vi "DPO_7K_Default Settings.vi"(8 "Error In":errorcluster, 11 "VISA resource name in":refnum<visa-resource-name>) -> (0 "error out":errorcluster, 3 "VISA resource name out":refnum<visa-resource-name>)   [LabVIEW 2020]
doc: "Establishes communication with the instrument and optionally performs an instrument identification query or an instrument reset. This VI also places the instrument in a default state needed for other instrument driver operations.\nRun this VI before running other instrument driver VIs for the instrument. You generally need to run the Initialize VI only once, at the beginning of an application."
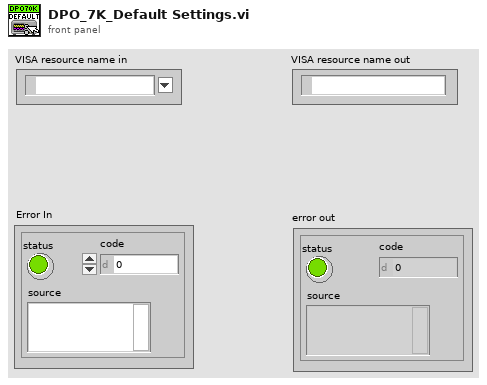
[diagram p1: front panel]
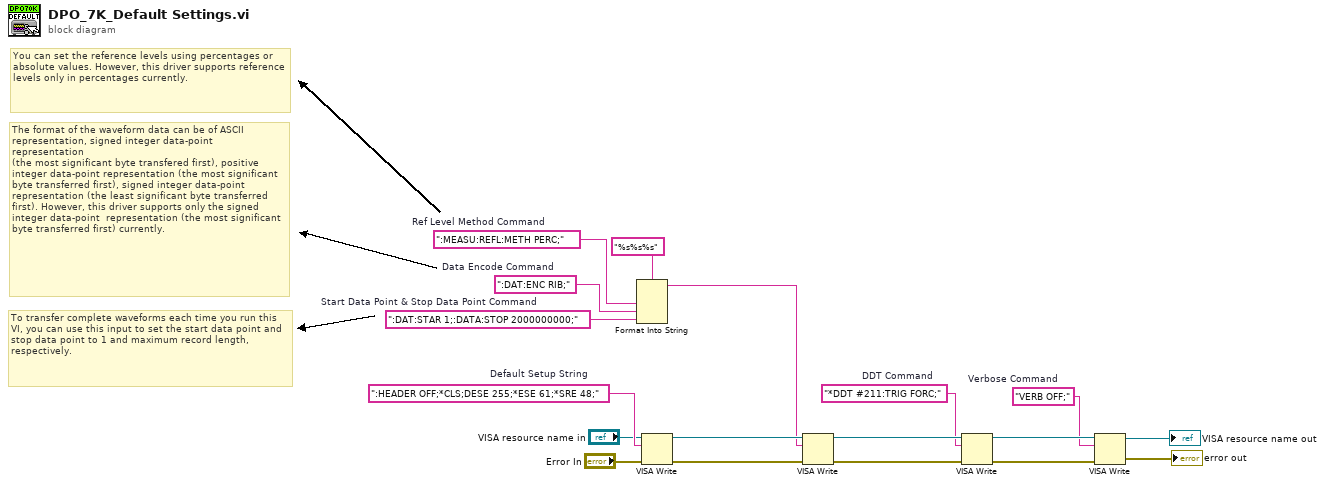
[diagram p0: block diagram]
diagram:
  w5 = ":DAT:STAR 1;:DATA:STOP 2000000000;"  # Start Data Point & Stop Data Point Command
  w6 = ":DAT:ENC RIB;"  # Data Encode Command
  w7 = ":HEADER OFF;*CLS;DESE 255;*ESE 61;*SRE 48;"  # Default Setup String
  w8 = "VERB OFF;"  # Verbose Command
  w11 = "*DDT #211:TRIG FORC;"  # DDT Command
  w18 = ":MEASU:REFL:METH PERC;"  # Ref Level Method Command
  # "To transfer complete waveforms each time you run this VI, you can use this input to set the start data point and stop data point to 1 and maximum record length, respectively."
  # "The format of the waveform data can be of ASCII\nrepresentation, signed integer data-point representation \n(the most significant byte transfered first), positive \ninteger data-point representation (the most significant \nbyte transferred first), signed integer data-point \nrepresentation (the least significant byte transferred first). However, this driver supports only the signed integer data-point  representation (the most significant byte transferred first) currently."
  # "You can set the reference levels using percentages or absolute values. However, this driver supports reference levels only in percentages currently."
  n1 = Format Into String(format string="%s%s%s", w18, w6, w5) -> (resulting string=w15:string)  [unwired: 2 in, 1 out]
  n2 = VISA Write(VISA resource name="VISA resource name in", write buffer=w7, error in (no error)="Error In") -> (VISA resource name out=w17:refnum<visa-resource-name>, error out=w16:errorcluster)  [unwired: 1 out]
  n3 = VISA Write(VISA resource name=w17, write buffer=w15, error in (no error)=w16) -> (VISA resource name out=w13:refnum<visa-resource-name>, error out=w12:errorcluster)  [unwired: 1 out]
  n4 = VISA Write(VISA resource name=w13, write buffer=w11, error in (no error)=w12) -> (VISA resource name out=w10:refnum<visa-resource-name>, error out=w9:errorcluster)  [unwired: 1 out]
  n5 = VISA Write(VISA resource name=w10, write buffer=w8, error in (no error)=w9) -> (VISA resource name out=→"VISA resource name out":refnum<visa-resource-name>, error out=→"error out":errorcluster)  [unwired: 1 out]
